vi "Read LHW-Data Objects.vi"(8 "error in (no error)":errorcluster, 11 "LHW-DataCollection in":refnum<class "LHW-DataCollection.lvclass">) -> (0 "error out":errorcluster, 2 "LHW-Data Objects":refnum<class "LHW-Data.lvclass">[](array[class]), 3 "LHW-DataCollection out":refnum<class "LHW-DataCollection.lvclass">)   [LabVIEW 2014, in "LHW-Data.lvlib" / "LHW-DataCollection.lvclass"]
doc: "Read LHW-DataObjects from Attribute."
uses:
  LHW-DataCollection.lvclass
  LHW-Data/LHW-Data.lvclass
  LHW-DataCollection.lvclass/LHW-DataCollection.ctl
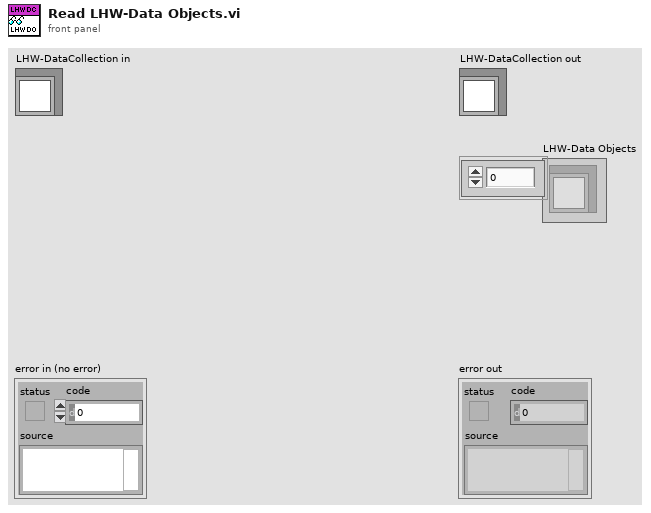
[diagram p1: front panel]
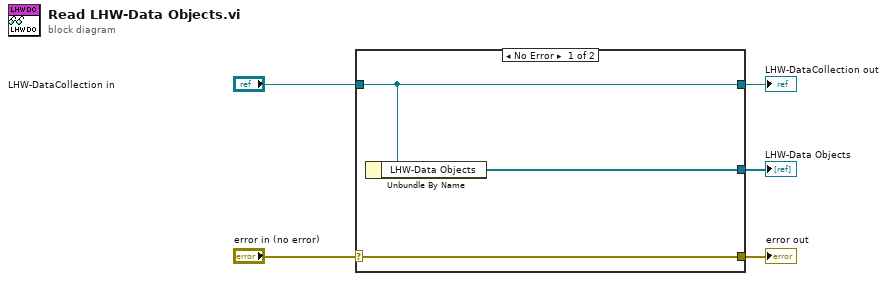
[diagram p0: block diagram]
diagram:
  n1 = case shown="No Error" "error in (no error)" {
    selector: "error in (no error)" -> [w8 w9]
    tunnel: [w8 w9] -> w4
    tunnel: [w7 w10] -> w2
    tunnel: "LHW-DataCollection in" -> [w7 w10]
    tunnel: [w6 _] -> w1
    frame No Error {
      n2 = Unbundle By Name(w7) -> ("LHW-Data Objects"=w6:refnum<class "LHW-Data.lvclass">[])
    }
    frame Error {
    }
  }
  "error out" <- w4
  "LHW-DataCollection out" <- w2
  "LHW-Data Objects" <- w1
